vi "oax_Open Tachless File.vi"(8 "error in":errorcluster) -> (0 "error out":errorcluster, 1 "Vibration File Path":path, 2 "Simulated Speed Profile Path (.ssp)":path, 3 "OK?":bool, 5 "Enum":T1(ring)=enum."Load tachless file")   [LabVIEW 2017]
panel:
  in  "Tachless Vibration File Path (.wav)":path
  in  "Simulated Speed Profile Path (.ssp)":path
  in  "OK":bool
  in  "Cancel":bool
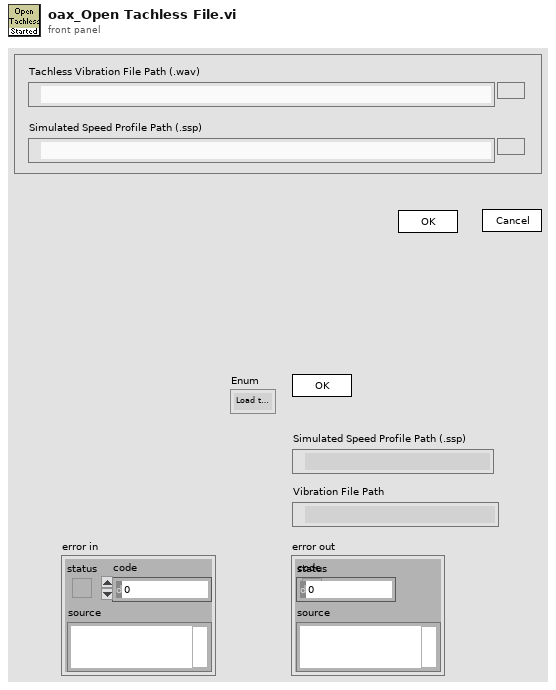
[diagram p1: front panel]
types:
  T1 = enum16{"Load .wav file", "Load .dat file", "Load tachless file", "Load .ssp file"}
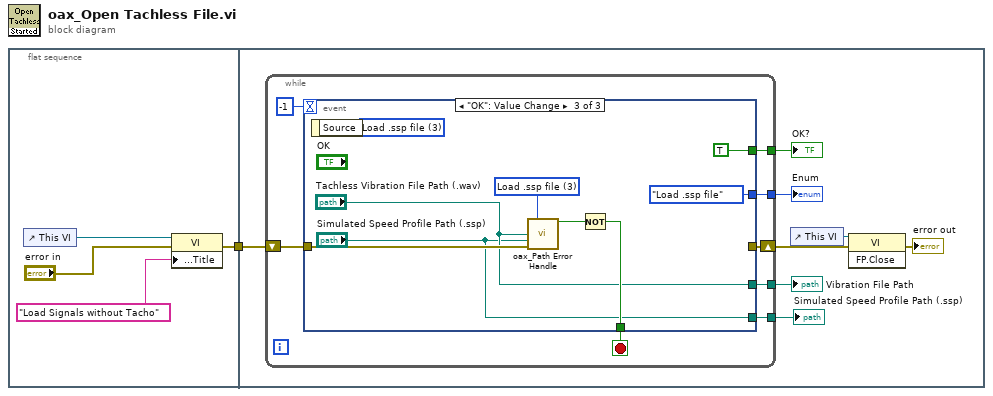
[diagram p0: block diagram]
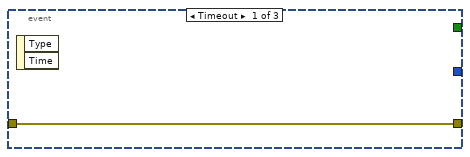
[diagram p2: hidden frame]
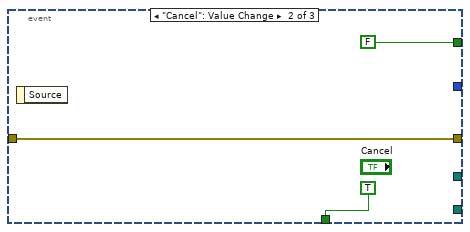
[diagram p3: hidden frame]
diagram:
  n1 = flat-sequence {
    tunnel: [w2] -> w1
    tunnel: w1 -> [w13]
    frame #0 {
      n2 = control-ref of="This VI"() -> (w5:refnum<vi>)
      n3 = property class="VI"(reference=w5, error in="error in", "Front Panel.Title"="Load Signals without Tacho" ("Front Panel Window:Title")) -> (error out=w2:errorcluster)  [unwired: 1 out]
    }
    frame #1 {
      n4 = while {
        shift-right: [w18] -> w10
        shift-left: w13 -> [w19]
        tunnel: [w17] -> w9
        tunnel: [w16] -> w8
        tunnel: [w15] -> w7
        tunnel: [w14] -> w6
        stop <- w20 stop-if-true
        n5 = event shown="[2] \"OK\": Value Change" {
          selector: _ -> [_ _ _]
          dyn-events: _ -> [_ _ _]
          timeout: -1 -> [_ _ _]
          tunnel: [_ TRUE w32] -> w20
          tunnel: w19 -> [w22 w24 w33]
          tunnel: [w22 w24 _] -> w18
          tunnel: [_ FALSE TRUE] -> w17
          tunnel: [_ _ "Tachless Vibration File Path (.wav)"] -> w16
          tunnel: [_ _ T1."Load .ssp file" ("Enum")] -> w15
          tunnel: [_ _ "Simulated Speed Profile Path (.ssp)"] -> w14
          event Timeout {
            n6 = event-data() -> ()  [unwired: 1 in, 2 out]
          }
          event "Cancel": Value Change {
            n7 = event-data() -> ()  [unwired: 1 in, 1 out]
          }
          event "OK": Value Change {
            (unwired) u16 3 items=["Load .wav file", "Load .dat file", "Load tachless file", "Load .ssp file"] ("Ring")
            w27 = u16 3 items=["Load .wav file", "Load .dat file", "Load tachless file", "Load .ssp file"] ("Ring")
            n8 = event-data() -> ()  [unwired: 1 in, 1 out]
            n9 = call <vilib>:"oax_Path Error Handle.vi"("Ring"=w27, "Vibration File Path (.wav)"="Tachless Vibration File Path (.wav)", "Simulated File Path (.ssp)"="Simulated Speed Profile Path (.ssp)", "error In"=w33) -> ("Error"=w28:bool)  [unwired: 10 in, 1 out]
            n10 = Not(x=w28) -> (.not. x?=w32:bool)
          }
        }
      }
      "Enum" <- w7
      "OK?" <- w9
      "Vibration File Path" <- w8
      "Simulated Speed Profile Path (.ssp)" <- w6
      n11 = control-ref of="This VI"() -> (w11:refnum<vi>)
      n12 = invoke class="VI" method="FP.Close"(reference=w11, error in=w10) -> (error out=→"error out":errorcluster)  [unwired: 1 in, 2 out]
    }
  }
